vi "MainUI.vi"() -> ()   [LabVIEW 2016]
uses:
  Controls/Operational Modes.ctl
  Controls/Shutter Manual.ctl
  Controls/Shutter States.ctl
  Controls/Flip Mirror Manual.ctl
  Controls/Lamps Manual.ctl
  Controls/Flip Mirrors.ctl
  Controls/Shutters.ctl
  Controls/Shutter Data.ctl
  Controls/Message Structure.ctl
panel:
  out "Quartz.Status":bool
  out "LED.Status":bool
  out "ThAr.Status 2":bool
  in  "Manual Lamp":T1
  in  "Solar Exp Time":dbl
  in  "ExtFlt Exp Time":dbl
  in  "LFCSim Exp Time":dbl
  in  "Sci Exp Time":dbl
  out "SimFlat.Time Stamp 2":timestamp format="%<%H:%M:%S%3u>T"
  out "ExtendedFlat.Time Stamp 2":timestamp format="%<%H:%M:%S%3u>T"
  out "Science.Time Stamp 2":timestamp format="%<%H:%M:%S%3u>T"
  out "LFCSim.Time Stamp 2":timestamp format="%<%H:%M:%S%3u>T"
  out "Solar.Time Stamp 3":timestamp format="%<%H:%M:%S%3u>T"
  out "SimFlat.Time Stamp":timestamp format="%<%H:%M:%S%3u>T"
  out "ExtendedFlat.Time Stamp":timestamp format="%<%H:%M:%S%3u>T"
  out "Science.Time Stamp":timestamp format="%<%H:%M:%S%3u>T"
  out "LFCSim.Time Stamp":timestamp format="%<%H:%M:%S%3u>T"
  out "Solar.Time Stamp":timestamp format="%<%H:%M:%S%3u>T"
  out "Solar.State":T2
  out "SimFlat.State":T2
  out "ExtendFlat.State":T2
  out "LFCSim.State":T2
  out "Science.State":T2
  out "Solar.Status":bool
  out "SimFlat.Status":bool
  out "ExtendFlat.Status":bool
  out "LFCSim.Status":bool
  out "Science.Status":bool
  in  "Manual Mirror":T3
  out "ThAr.Time Stamp":timestamp format="%<%H:%M:%S%3u>T"
  out "ThAr.Status":bool caption="ThAr"
  out "ExtFlat.Time Stamp":timestamp format="%<%H:%M:%S%3u>T"
  out "Solar.Time Stamp 2":timestamp format="%<%H:%M:%S%3u>T"
  out "Solar.Status 2":bool caption="Solar"
  out "ExtFlat.Status":bool caption="ExtFlat"
  out "Remaining":dbl
  in  "SimFlt Exp Time":dbl
  in  "stop":bool
  in  "Manual Trigger":bool
  in  "Manual Shutter":T4
  in  "EXPRES Mode":T5
  # "Timeouts"
  # "Shutter States"
  # "Open"
  # "Close"
  # "Science"
  # "Sim LFC"
  # "Ext Flat"
  # "Sim Flat"
  # "Solar"
  # "Flip Mirrors"
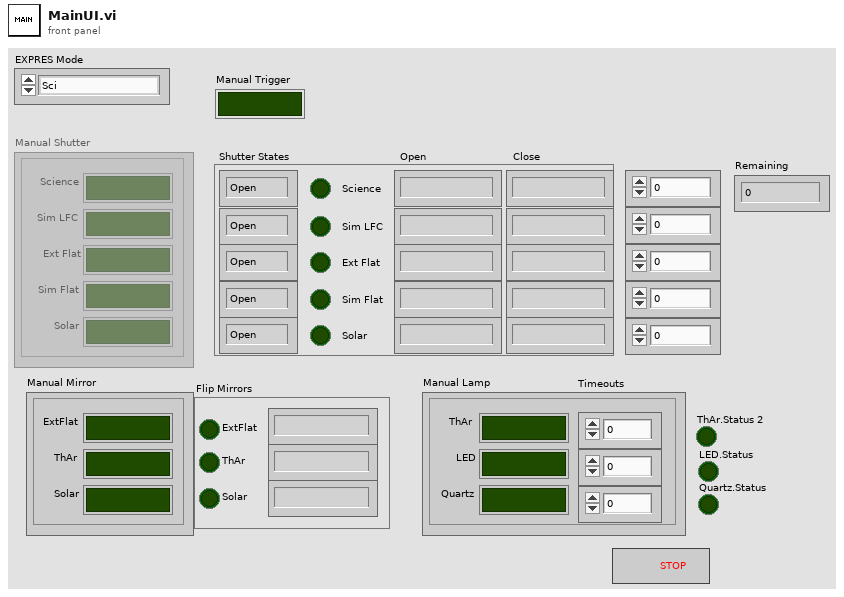
[diagram p1: front panel]
types:
  T1 = typedef "Lamps Manual.ctl" = cluster{"ThAr":bool, "Quartz":bool, "LED":bool, "ThAr Timeout":dbl, "LED Timeout":dbl, "Quartz Timeout":dbl}
  T2 = typedef "Shutter States.ctl" = enum16{"Open", "Close", "Wait", "Off", "Arm", "Idle"}
  T3 = typedef "Flip Mirror Manual.ctl" = cluster{"ExtFlat":bool, "Solar":bool, "ThAr":bool}
  T4 = typedef "Shutter Manual.ctl" = cluster{"Science":bool, "Solar":bool, "Ext Flat":bool, "Sim LFC":bool, "Sim Flat":bool}
  T5 = typedef "Operational Modes.ctl" = enum16{"Sci", "Sci-LFC", "Solar", "Solar-LFC", "LFC", "LFC-Sim", "LFC-Both", "ThAr", "ThAr-LFC", "Flat", "ExtFlat", "ExtFlat-Sim", "ExtFlat-Both", "Qtz", "ExtQtz", "ExtQtz-Sim", "ExtQtz-Both", "Dark", "Manual", "Off"}
  T6 = enum8{"Enabled", "Disabled", "Disabled and Grayed Out"}
  T7 = typedef "Message Structure.ctl" = cluster{"Data":variant, "Cmd":string}
  T8 = typedef "Shutters.ctl" = cluster{"Science":T9, "LFCSim":T9, "ExtendFlat":T9, "SimFlat":T9, "Solar":T9}
  T9 = typedef "Shutter Data.ctl" = cluster{"Status":bool, "State":T2, "Time Stamps":cluster{"Open":timestamp, "Close":timestamp}}
  T10 = typedef "Flip Mirrors.ctl" = cluster{"Solar":cluster{"Status":bool, "Time Stamp":timestamp}, "ExtFlat":cluster{"Status":bool, "Time Stamp":timestamp}, "ThAr":cluster{"Status":bool, "Time Stamp":timestamp}}
  T11 = cluster{"ThAr":cluster{"Time Stamp":timestamp, "Status":bool, "Timeout":dbl}, "LED":cluster{"Time Stamp":timestamp, "Status":bool, "Timeout":dbl}, "Quartz":cluster{"Time Stamp":timestamp, "Status":bool, "Timeout":dbl}}
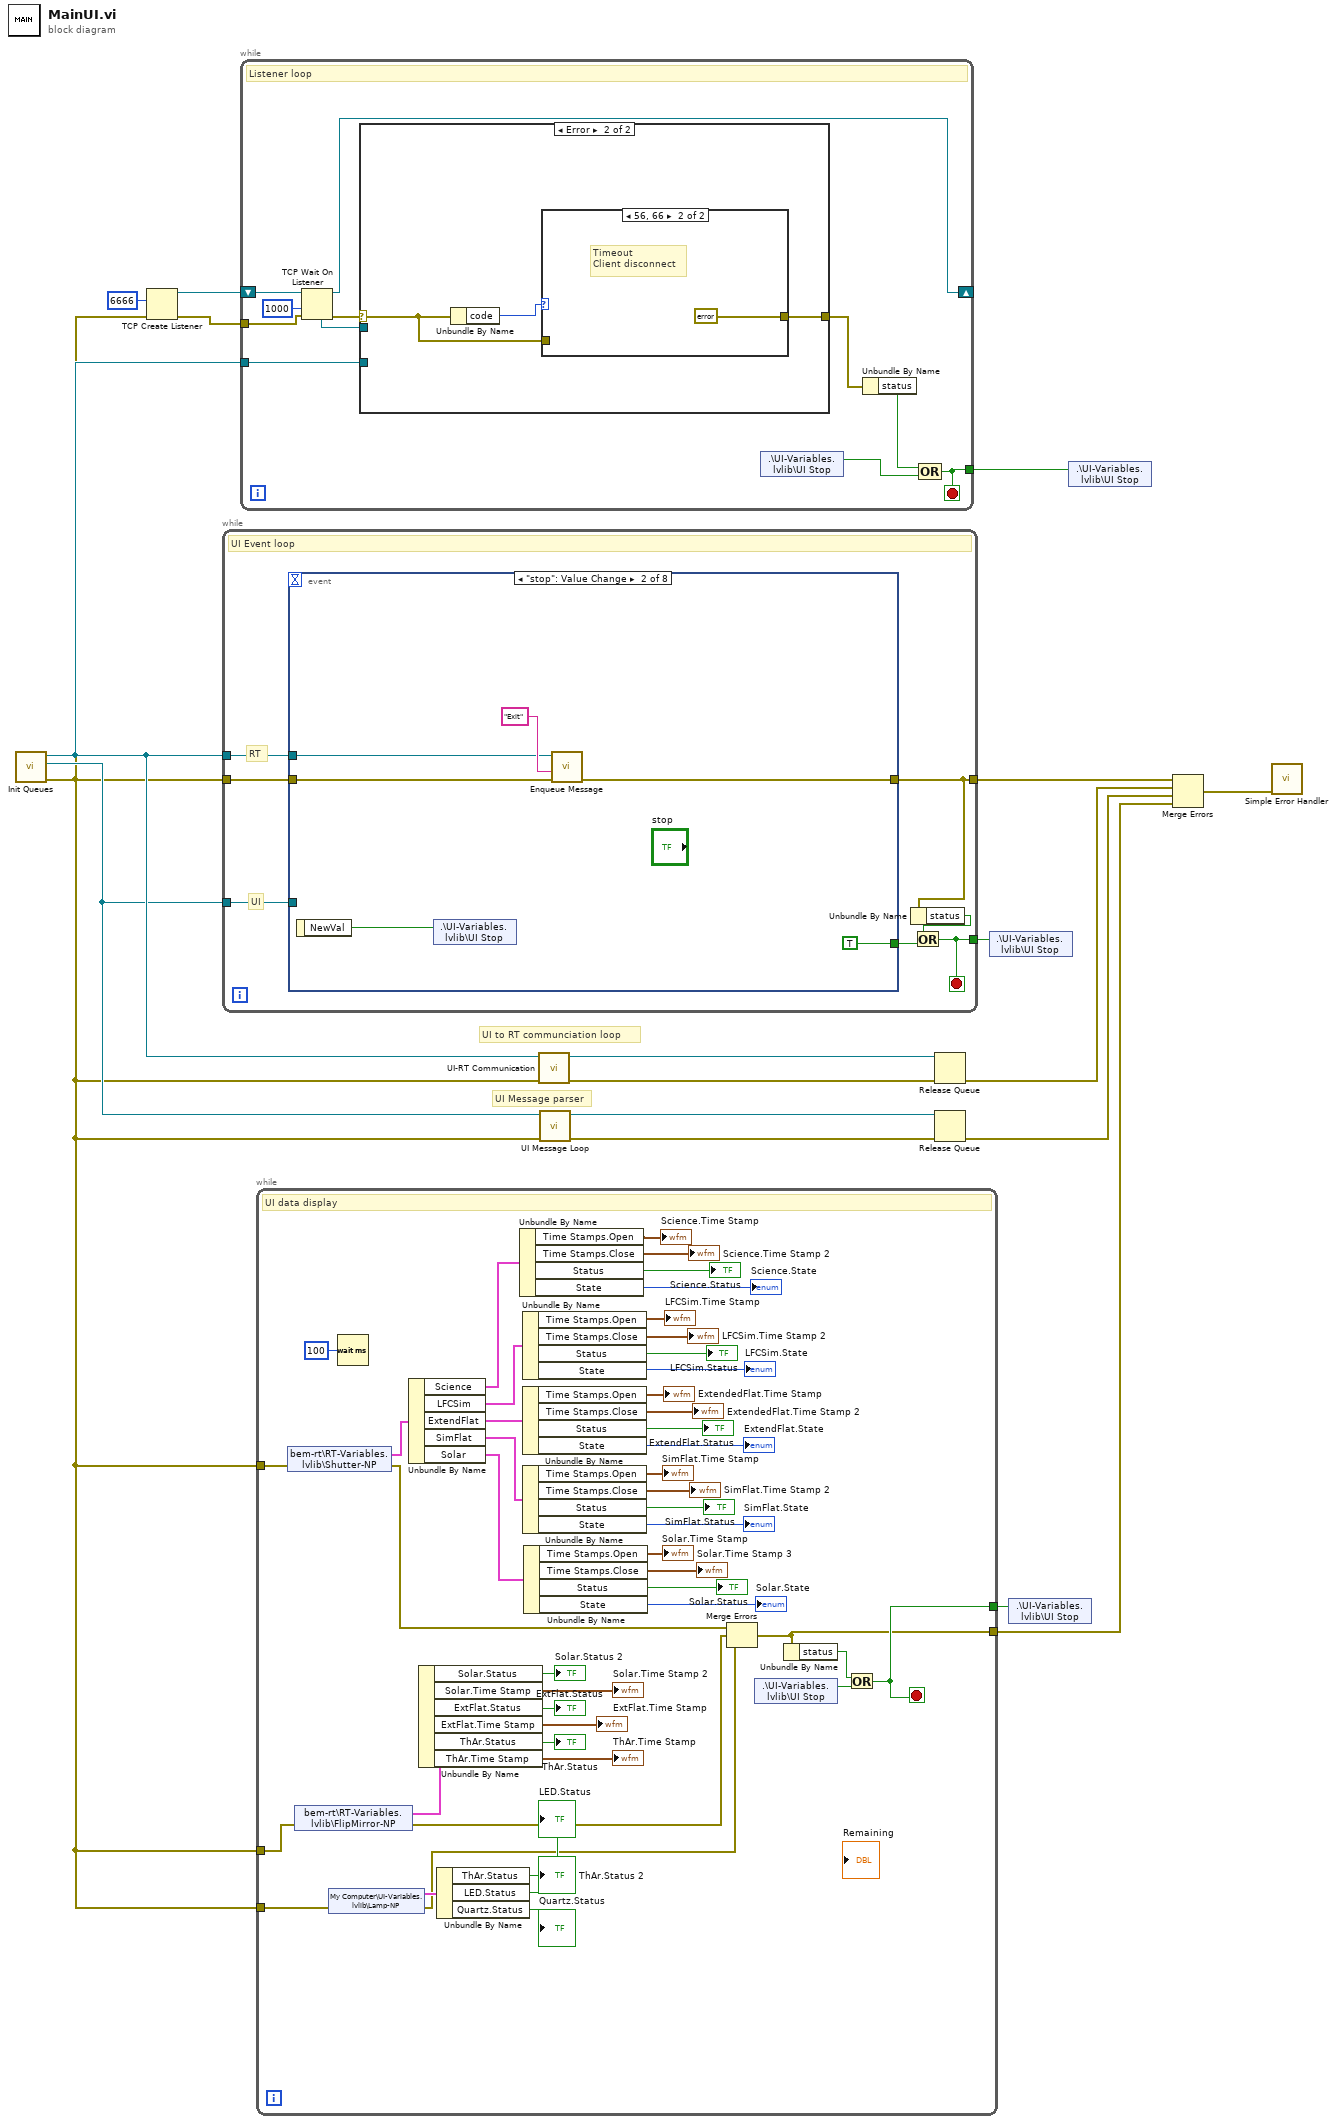
[diagram p0: block diagram]
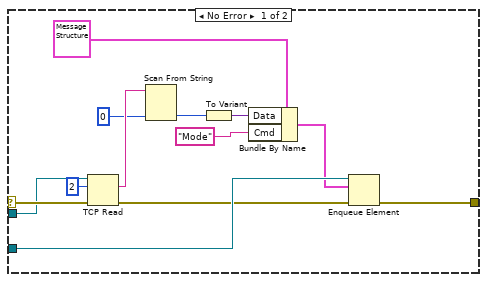
[diagram p2: hidden frame]
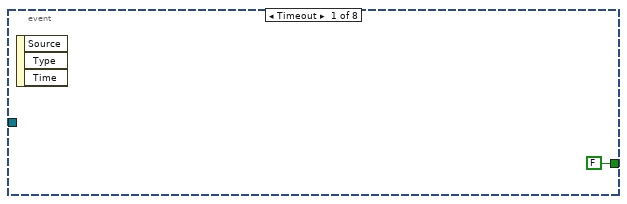
[diagram p4: hidden frame]
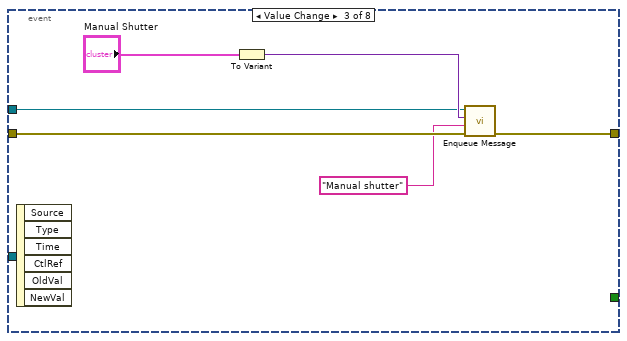
[diagram p5: hidden frame]
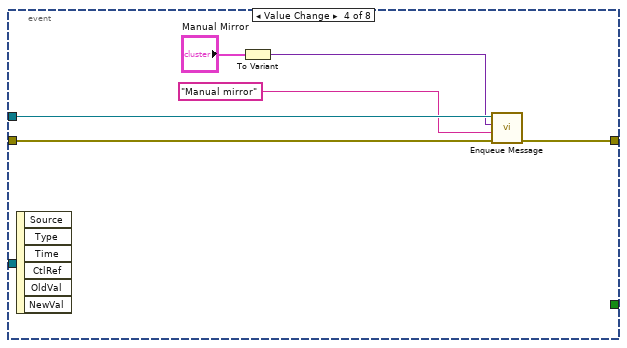
[diagram p6: hidden frame]
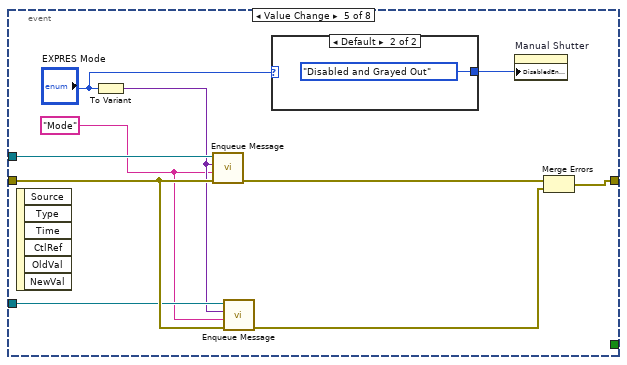
[diagram p7: hidden frame]
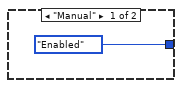
[diagram p8: hidden frame]
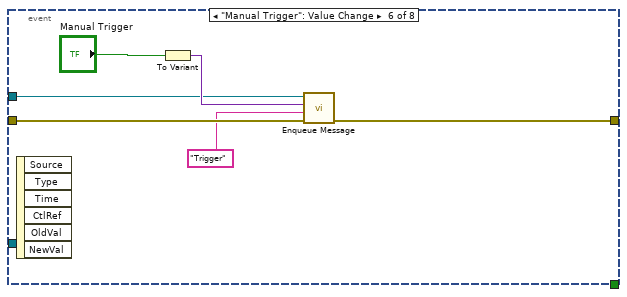
[diagram p9: hidden frame]
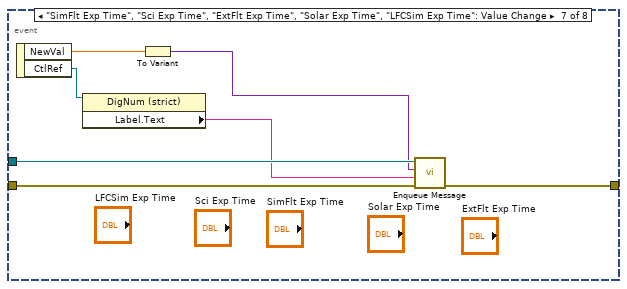
[diagram p10: hidden frame]
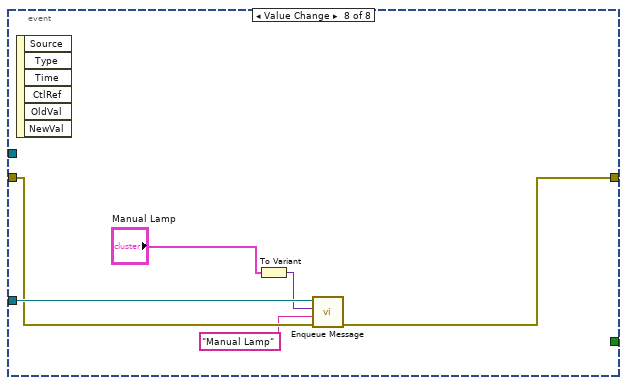
[diagram p11: hidden frame]
diagram:
  # "UI Message parser"
  # "UI to RT communciation loop"
  n1 = call "Init Queues.vi"() -> ("error out"=w1:errorcluster, "UI Queue"=w7:refnum<queue>, "UI-RT Queue"=w10:refnum<queue>)  [unwired: 9 in]
  n2 = TCP Create Listener(8:w1, 10:u16 6666 ("port")) -> (0:w12:errorcluster, 3:w13:refnum<k5>)  [unwired: 3 in, 1 out]
  n3 = while {
    tunnel: w10 -> [w25]
    tunnel: w1 -> [w24]
    tunnel: [w20] -> w16
    tunnel: [w23] -> w18
    tunnel: w7 -> [w19]
    stop <- w23 stop-if-true
    # "UI"
    # "RT"
    # "UI Event loop"
    n4 = event shown="[1] \"stop\": Value Change" {
      selector: _ -> [_ _ _ _ _ _ _ _]
      dyn-events: _ -> [_ _ _ _ _ _ _ _]
      timeout: _ -> [_ _ _ _ _ _ _ _]
      tunnel: [FALSE TRUE _ _ _ _ _ _] -> w22
      tunnel: w25 -> [_ w29 w34 w41 w52 w57 w67 _]
      tunnel: w24 -> [_ w28 w37 w42 w51 w61 w66 w74]
      tunnel: [_ w27 w36 w43 w46 w60 w65 w73] -> w20
      tunnel: w19 -> [_ _ _ _ w50 _ _ w75]
      event Timeout {
        n5 = event-data() -> ()  [unwired: 1 in, 3 out]
      }
      event "stop": Value Change {
        n6 = event-data() -> ("NewVal"=w31:bool)  [unwired: 1 in]
        n7 = shared-variable ".\\UI-Variables.lvlib\\UI Stop"(w31) -> ()  [unwired: 1 in, 1 out]
        n8 = call "Enqueue Message.vi"("error in (no error)"=w28, "Cmd"="Exit", "Queue In"=w29) -> ("error out"=w27:errorcluster)  [unwired: 8 in]
      }
      event Value Change {
        n9 = event-data() -> ()  [unwired: 1 in, 6 out]
        n10 = To Variant(anything="Manual Shutter") -> (Variant=w35:variant)
        n11 = call "Enqueue Message.vi"("error in (no error)"=w37, "Cmd"="Manual shutter", "Data variant"=w35, "Queue In"=w34) -> ("error out"=w36:errorcluster)  [unwired: 7 in]
      }
      event Value Change {
        n12 = event-data() -> ()  [unwired: 1 in, 6 out]
        n13 = To Variant(anything="Manual Mirror") -> (Variant=w40:variant)
        n14 = call "Enqueue Message.vi"("error in (no error)"=w42, "Cmd"="Manual mirror", "Data variant"=w40, "Queue In"=w41) -> ("error out"=w43:errorcluster)  [unwired: 7 in]
      }
      event Value Change {
        w48 = "Mode"
        n15 = event-data() -> ()  [unwired: 1 in, 6 out]
        n16 = To Variant(anything="EXPRES Mode") -> (Variant=w49:variant)
        n17 = call "Enqueue Message.vi"("error in (no error)"=w51, "Cmd"=w48, "Data variant"=w49, "Queue In"=w52) -> ("error out"=w47:errorcluster)  [unwired: 7 in]
        n18 = call "Enqueue Message.vi"("error in (no error)"=w51, "Cmd"=w48, "Data variant"=w49, "Queue In"=w50) -> ("error out"=w45:errorcluster)  [unwired: 7 in]
        n19 = case shown="Default" "EXPRES Mode" {
          tunnel: [T6."Enabled" ("Disabled") T6."Disabled and Grayed Out" ("Disabled")] -> w54
          frame "Manual" {
          }
          frame Default {
          }
        }
        n20 = property on="Manual Shutter" class="Clust (strict)"("DisabledEnum"=w54) -> ()  [unwired: 2 in, 2 out]
        n21 = Merge Errors(w47, w45) -> (w46:errorcluster)
      }
      event "Manual Trigger": Value Change {
        n22 = event-data() -> ()  [unwired: 1 in, 6 out]
        n23 = To Variant(anything="Manual Trigger") -> (Variant=w58:variant)
        n24 = call "Enqueue Message.vi"("error in (no error)"=w61, "Cmd"="Trigger", "Data variant"=w58, "Queue In"=w57) -> ("error out"=w60:errorcluster)  [unwired: 7 in]
      }
      event "SimFlt Exp Time", "Sci Exp Time", "ExtFlt Exp Time", "Solar Exp Time", "LFCSim Exp Time": Value Change {
        n25 = event-data() -> ("NewVal"=w69:dbl, "CtlRef"=w68:refnum<vi>)  [unwired: 1 in]
        n26 = property class="DigNum (strict)"(reference=w68) -> ("Label.Text"=w63:string)  [unwired: 1 in, 2 out]
        n27 = To Variant(anything=w69) -> (Variant=w64:variant)
        n28 = call "Enqueue Message.vi"("error in (no error)"=w66, "Cmd"=w63, "Data variant"=w64, "Queue In"=w67) -> ("error out"=w65:errorcluster)  [unwired: 7 in]
      }
      event Value Change {
        n29 = event-data() -> ()  [unwired: 1 in, 6 out]
        n30 = To Variant(anything="Manual Lamp") -> (Variant=w70:variant)
        n31 = call "Enqueue Message.vi"("error in (no error)"=w74, "Cmd"="Manual Lamp", "Data variant"=w70, "Queue In"=w75) -> ("error out"=w73:errorcluster)  [unwired: 7 in]
      }
    }
    n32 = Unbundle By Name(w20) -> ("status"=w21:bool)
    n33 = Or(x=w21, y=w22) -> (x .or. y?=w23:bool)
  }
  n34 = while {
    tunnel: [w85] -> w14
    tunnel: w12 -> [w79]
    tunnel: w10 -> [w78]
    shift-right: [w77] -> _
    shift-left: w13 -> [w83]
    stop <- w85 stop-if-true
    # "Listener loop"
    n35 = TCP Wait On Listener(8:w79, 9:1000 ("timeout ms (wait forever: -1)"), 11:w83) -> (0:w81:errorcluster, 3:w77:refnum<k5>, 4:w76:refnum<k5>)  [unwired: 1 in, 2 out]
    n36 = case shown="Error" w81 {
      selector: w81 -> [w97 w101]
      tunnel: [w99 w100] -> w80
      tunnel: w78 -> [w98 _]
      tunnel: w76 -> [w96 _]
      frame No Error {
        n37 = TCP Read(connection ID=w96, bytes to read=2, error in (no error)=w97) -> (data out=w94:string, error out=w87:errorcluster)  [unwired: 2 in, 1 out]
        n38 = Scan From String(input string=w94, default 1=u32 0) -> (output 1=w88:u32)  [unwired: 3 in, 3 out]
        n39 = To Variant(anything=w88) -> (Variant=w92:variant)
        n40 = Bundle By Name(cluster=T7 {"Data"=variant, "Cmd"=""}, "Data"=w92, "Cmd"="Mode") -> (w89:T7)
        n41 = Enqueue Element(queue=w98, element=w89, error in (no error)=w87) -> (error out=w99:errorcluster)  [unwired: 1 in, 2 out]
      }
      frame Error {
        n42 = Unbundle By Name(w101) -> ("code"=w102:i32)
        n43 = case shown="56, 66" w102 {
          tunnel: w101 -> [w103 _]
          tunnel: [w103 errorcluster {"status"=FALSE, "code"=0, "source"=""} ("error constant")] -> w100
          frame 0, Default {
          }
          frame 56, 66 {
            # "Timeout\nClient disconnect"
          }
        }
      }
    }
    n44 = shared-variable ".\\UI-Variables.lvlib\\UI Stop"() -> (w86:bool)  [unwired: 1 in, 1 out]
    n45 = Unbundle By Name(w80) -> ("status"=w84:bool)
    n46 = Compound Arithmetic op=OR(w84, w86) -> (w85:bool)
  }
  n47 = while {
    tunnel: w1 -> [w148]
    tunnel: [w150] -> w15
    tunnel: [w128] -> w3
    tunnel: w1 -> [w131]
    tunnel: w1 -> [w106]
    stop <- w150 stop-if-true
    # "UI data display"
    n48 = shared-variable "bem-rt\\RT-Variables.lvlib\\Shutter-NP"(error in=w148) -> (w147:T8, error out=w129:errorcluster)
    n49 = shared-variable "bem-rt\\RT-Variables.lvlib\\FlipMirror-NP"(error in=w131) -> (w127:T10, error out=w130:errorcluster)
    n50 = shared-variable "My Computer\\UI-Variables.lvlib\\Lamp-NP"(error in=w106) -> (w110:T11, error out=w105:errorcluster)
    n51 = Wait (ms)(milliseconds to wait=u32 100) -> ()  [unwired: 1 out]
    n52 = Unbundle By Name(w147) -> ("Science"=w146:T9, "LFCSim"=w145:T9, "ExtendFlat"=w140:T9, "SimFlat"=w139:T9, "Solar"=w138:T9)
    n53 = Unbundle By Name(w127) -> ("Solar.Status"=→"Solar.Status 2":bool, "Solar.Time Stamp"=→"Solar.Time Stamp 2":timestamp, "ExtFlat.Status"=→"ExtFlat.Status":bool, "ExtFlat.Time Stamp"=→"ExtFlat.Time Stamp":timestamp, "ThAr.Status"=→"ThAr.Status":bool, "ThAr.Time Stamp"=→"ThAr.Time Stamp":timestamp)
    n54 = Unbundle By Name(w110) -> ("ThAr.Status"=→"ThAr.Status 2":bool, "LED.Status"=→"LED.Status":bool, "Quartz.Status"=→"Quartz.Status":bool)
    n55 = Unbundle By Name(w146) -> ("Time Stamps.Open"=→"Science.Time Stamp":timestamp, "Time Stamps.Close"=→"Science.Time Stamp 2":timestamp, "Status"=→"Science.Status":bool, "State"=→"Science.State":T2)
    n56 = Unbundle By Name(w145) -> ("Time Stamps.Open"=→"LFCSim.Time Stamp":timestamp, "Time Stamps.Close"=→"LFCSim.Time Stamp 2":timestamp, "Status"=→"LFCSim.Status":bool, "State"=→"LFCSim.State":T2)
    n57 = Unbundle By Name(w140) -> ("Time Stamps.Open"=→"ExtendedFlat.Time Stamp":timestamp, "Time Stamps.Close"=→"ExtendedFlat.Time Stamp 2":timestamp, "Status"=→"ExtendFlat.Status":bool, "State"=→"ExtendFlat.State":T2)
    n58 = Unbundle By Name(w139) -> ("Time Stamps.Open"=→"SimFlat.Time Stamp":timestamp, "Time Stamps.Close"=→"SimFlat.Time Stamp 2":timestamp, "Status"=→"SimFlat.Status":bool, "State"=→"SimFlat.State":T2)
    n59 = Unbundle By Name(w138) -> ("Time Stamps.Open"=→"Solar.Time Stamp":timestamp, "Time Stamps.Close"=→"Solar.Time Stamp 3":timestamp, "Status"=→"Solar.Status":bool, "State"=→"Solar.State":T2)
    n60 = Merge Errors(w129, w130, w105) -> (w128:errorcluster)
    n61 = shared-variable ".\\UI-Variables.lvlib\\UI Stop"() -> (w151:bool)  [unwired: 1 in, 1 out]
    n62 = Unbundle By Name(w128) -> ("status"=w149:bool)
    n63 = Or(x=w149, y=w151) -> (x .or. y?=w150:bool)
  }
  n64 = call "UI-RT Communication.vi"("error in (no error)"=w1, "UI-RT Queue In"=w10) -> ("error out"=w6:errorcluster, "UI-RT Queue Out"=w17:refnum<queue>)  [unwired: 8 in]
  n65 = call "UI Message Loop.vi"("error in (no error)"=w1, "UI Queue In"=w7) -> ("error out"=w9:errorcluster, "UI Queue Out"=w8:refnum<queue>)  [unwired: 8 in]
  n66 = Release Queue(queue=w17, error in (no error)=w6) -> (error out=w5:errorcluster)  [unwired: 1 in, 2 out]
  n67 = Release Queue(queue=w8, error in (no error)=w9) -> (error out=w4:errorcluster)  [unwired: 1 in, 2 out]
  n68 = shared-variable ".\\UI-Variables.lvlib\\UI Stop"(w18) -> ()  [unwired: 1 in, 1 out]
  n69 = shared-variable ".\\UI-Variables.lvlib\\UI Stop"(w15) -> ()  [unwired: 1 in, 1 out]
  n70 = shared-variable ".\\UI-Variables.lvlib\\UI Stop"(w14) -> ()  [unwired: 1 in, 1 out]
  n71 = Merge Errors(w16, w5, w4, w3) -> (w2:errorcluster)
  n72 = call <vilib>:"Simple Error Handler.vi"("error in (no error)"=w2) -> ()  [unwired: 4 in, 5 out]
